vi "SetClassQueue.vi"(8 "ErrorIn(No Error)":errorcluster caption="entrée d'erreur (pas d'erreur)", 11 "DefaultDev.lvclass":refnum<class "LSCI332.lvclass">) -> (0 "sortie d'erreur":errorcluster, 3 "DefaultDev.lvclass Out":refnum<class "LSCI332.lvclass">)   [LabVIEW 2012, in "LSCI332.lvclass"]
uses:
  LSCI332.lvclass
  BaseDevice/BaseDevice.lvclass
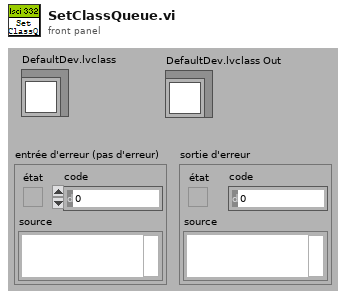
[diagram p1: front panel]
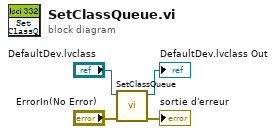
[diagram p0: block diagram]
diagram:
  n1 = call-parent "SetClassQueue.vi"("ErrorIn(No Error)"="ErrorIn(No Error)", "BaseDevice.lvclass"="DefaultDev.lvclass") -> ("sortie d'erreur"=→"sortie d'erreur":errorcluster, "BaseDevice.lvclass Out"=→"DefaultDev.lvclass Out":refnum<class "LSCI332.lvclass">)  [unwired: 8 in]
